vi "QDMH Check Error.vi"(7 "Filtered Error Codes":i32[](array[numeric]), 8 "error in (no error)":errorcluster, 10 "Case":string, 11 "queue":refnum<queue>) -> (0 "error out":errorcluster, 3 "queue out":refnum<queue>)   [LabVIEW 2019]
doc: "This VI is part of the QDMH template. It checks the error code to see if a non-filtered error has occured. If it has, it will place the Error case on the queue and add the pertinent information to the data variant. It will also clear the error.\n\nAAL 9/09"
uses:
  QDMH Poly VIs/QDMH POLY Enqueue Cluster.vi
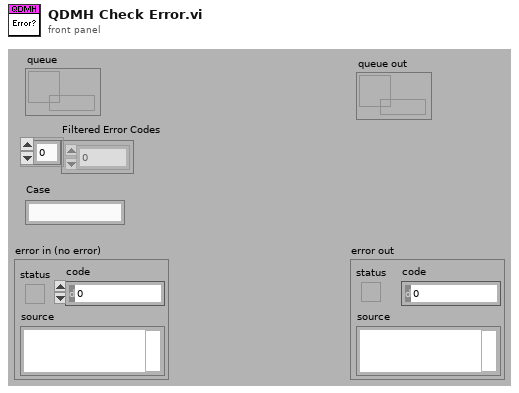
[diagram p1: front panel]
types:
  T1 = cluster{"Case":string, "error in (no error)":errorcluster}
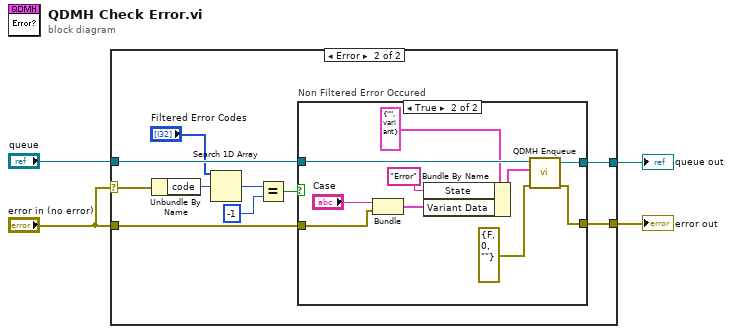
[diagram p0: block diagram]
diagram:
  n1 = case shown="Error" "error in (no error)" {
    selector: "error in (no error)" -> [_ w12]
    tunnel: "queue" -> [w6 w16]
    tunnel: [w6 w15] -> w3
    tunnel: "error in (no error)" -> [w5 w14]
    tunnel: [w5 w13] -> w2
    frame No Error {
    }
    frame Error {
      n2 = Unbundle By Name(w12) -> ("code"=w11:i32)
      n3 = Search 1D Array(1D array="Filtered Error Codes", element=w11) -> (index of element=w9:i32)  [unwired: 1 out]
      n4 = Equal?(x=w9, y=-1) -> (x = y?=w7:bool)
      n5 = case "Non Filtered Error Occured" shown="True" w7 {
        tunnel: w16 -> [w18 w28]
        tunnel: [w18 w27] -> w15
        tunnel: w14 -> [w17 w21]
        tunnel: [w17 w19] -> w13
        frame False {
        }
        frame True {
          n6 = Bundle("Case"="Case", "error in (no error)"=w21) -> (w23:T1)  [unwired: 1 out]
          n7 = Bundle By Name(cluster=cluster{"State":string, "Variant Data":variant} {"State"="", "Variant Data"=variant} ("QDSM Element"), "State"="Error", "Variant Data"=w23) -> (w24:cluster{"State":string, "Variant Data":variant})
          n8 = call-poly "QDMH Enqueue.vi"("error in (no error)"=errorcluster {"status"=FALSE, "code"=0, "source"=""}, "QDSM Element"=w24, "queue"=w28) -> ("error out"=w19:errorcluster, "queue out"=w27:refnum<queue>)  [unwired: 7 out]
        }
      }
    }
  }
  "queue out" <- w3
  "error out" <- w2
